vi "ukol2.vi"() -> ()   [LabVIEW 2023]
uses:
  <vilib>/Analysis/4window.llb/windowTd.ctl
  <vilib>/Waveform/WDTOps.llb/WDT Get Waveform Subset DBL.vi
  <vilib>/measure/maspectr.llb/FFT Spectrum (Mag-Phase) for 1 Chan.vi
  <vilib>/addons/Time Frequency Analysis/Transform.llb/TFA STFT (Waveform).vi
  <vilib>/Analysis/NI_AALBase.lvlib
  <vilib>/addons/_Advanced Signal Processing/NI_AdvSigProcTFA.lvlib
  <vilib>/measure/NI_MAPro.lvlib
  <vilib>/Analysis/NI_AALPro.lvlib
panel:
  out "1/x":dbl
  out "df":dbl
  out "Waveform Graph 2":cluster{"f0":dbl, "df":dbl, "magnitude":dbl[]}[](graph)
  out "Coefficients 2":dbl[][](graph)
  out "Coefficients":dbl[][](graph)
  in  "time-frequency sampling info":cluster{"time steps":i32, "frequency bins":i32}={"time steps"=-1, "frequency bins"=512}
  out "Waveform Graph":waveform(dbl)(graph)
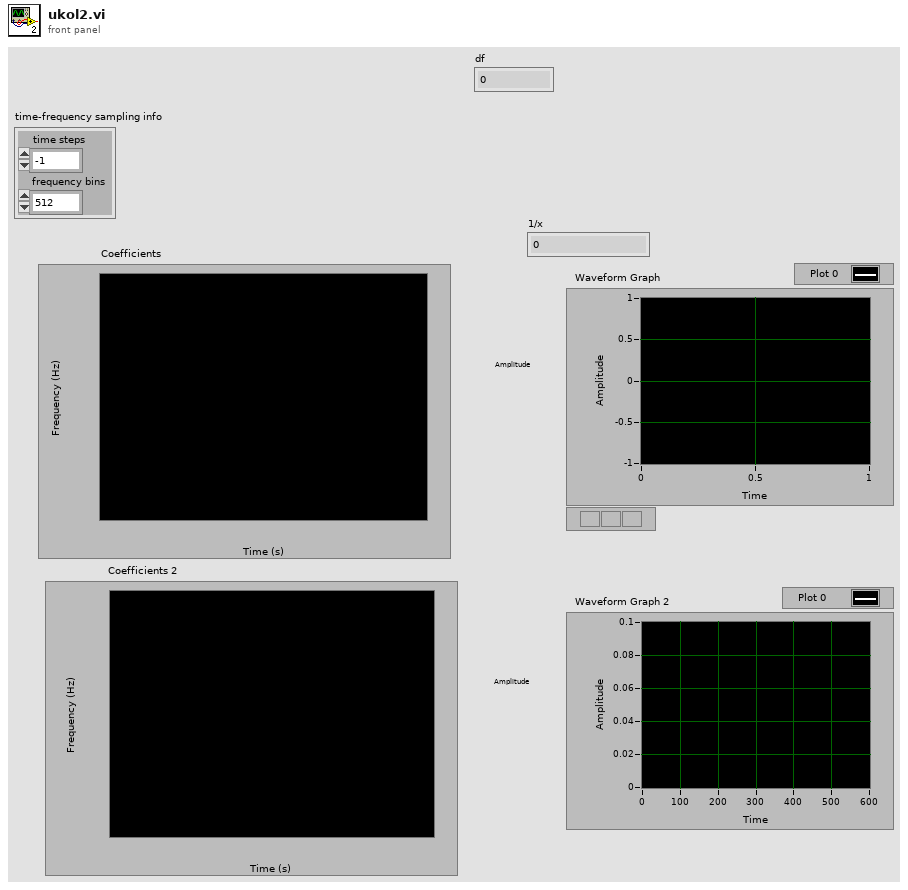
[diagram p1: front panel]
types:
  T1 = typedef "NI_AALPro.lvlib/windowTd.ctl" = u32
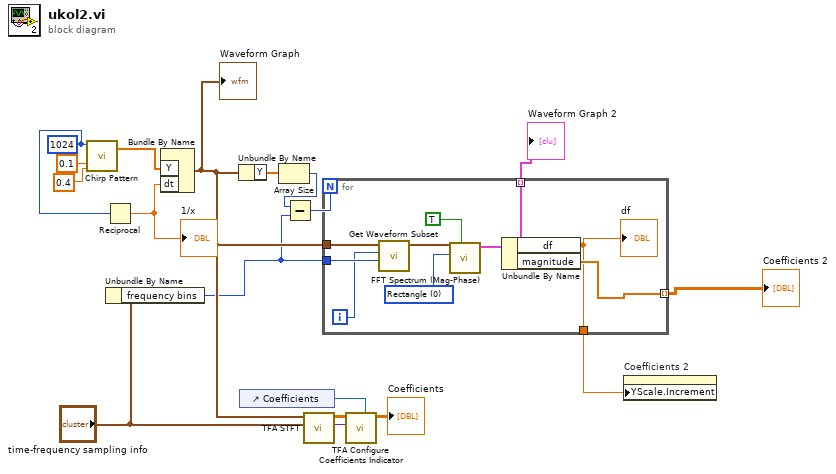
[diagram p0: block diagram]
diagram:
  w15 = 1024 ("samples")
  n1 = call <vilib>:"Chirp Pattern.vi"("f2"=0.4, "f1"=0.1, "samples"=w15) -> ("Chirp Pattern"=w16:dbl[])  [unwired: 1 in, 1 out]
  n2 = Reciprocal(x=w15) -> (1/x=w14:dbl)
  "1/x" <- w14
  n3 = Unbundle By Name("time-frequency sampling info") -> ("frequency bins"=w6:i32)
  n4 = Bundle By Name("Y"=w16, "dt"=w14) -> (w9:waveform(dbl))  [unwired: 1 in]
  "Waveform Graph" <- w9
  n5 = Unbundle By Name(w9) -> ("Y"=w8:dbl[])
  n6 = control-ref of="Coefficients"() -> (w13:refnum<vi>)
  n7 = Array Size(array=w8) -> (size(s)=w7:i32)
  n8 = Subtract(x=w7, y=w6) -> (x-y=w5:i32)
  n9 = call-poly <vilib>:"TFA STFT.vi"("time-frequency sampling info"="time-frequency sampling info", "signal"=w9) -> ("scale info"=w3:variant, "STFT coef"=w11:cdb[][])  [unwired: 7 in, 1 out]
  n10 = for {
    N: w5 -> [_]
    tunnel: w6 -> [w27]
    tunnel: w9 -> [w26]
    tunnel: [w21] -> w1 mode=indexing
    tunnel: [w19] -> w4 mode=indexing
    tunnel: [w20] -> w2
    i -> [w24]
    w22 = T1 0 items=["Rectangle"=0, "Hanning"=1, "Hamming"=2, "Blackman-Harris"=3, "Exact Blackman"=4, "Blackman"=5, "Flat Top"=6, "4 Term B-Harris "=7, "7 Term B-Harris"=8, "Low Sidelobe"=9, "Blackman Nuttall"=11, "Triangle"=30, "Bartlett-Hanning"=31, "Bohman"=32, "Parzen"=33, "Welch"=34, "Kaiser"=60, "Dolph-Chebyshev"=61, "Gaussian"=62] ("window")
    n11 = call-poly <vilib>:"Get Waveform Subset.vi"("duration"=w27, "start samples/time"=w24, "waveform in"=w26) -> ("waveform out"=w25:waveform(dbl))  [unwired: 3 in, 3 out]
    n12 = call-poly <vilib>:"FFT Spectrum (Mag-Phase).vi"("restart averaging (F)"=TRUE, "window"=w22, "time signal"=w25) -> ("magnitude"=w19:cluster{"f0":dbl, "df":dbl, "magnitude":dbl[]})  [unwired: 4 in, 4 out]
    n13 = Unbundle By Name(w19) -> ("df"=w20:dbl, "magnitude"=w21:dbl[])
    "df" <- w20
  }
  "Coefficients 2" <- w1
  "Waveform Graph 2" <- w4
  n14 = call <vilib>:"TFA Configure Coefficients Indicator.vi"("reference of TF coefficients indicator"=w13, "scale info"=w3, "TF coefficients"=w11) -> ("TF coefficients indicator"=→"Coefficients":dbl[][])  [unwired: 4 in, 4 out]
  n15 = property on="Coefficients 2" class="IntGraph (strict)"("YScale.Increment"=w2) -> ()  [unwired: 2 in, 2 out]
